vi "Close.vi"(8 "error in (no error)":errorcluster, 11 "CSV in":refnum<class "CSV.lvclass">) -> (0 "error out":errorcluster, 3 "CSV out":refnum<class "CSV.lvclass">)   [LabVIEW 2014, in "CSV.lvclass"]
uses:
  CSV.lvclass
  Report/Report.lvclass
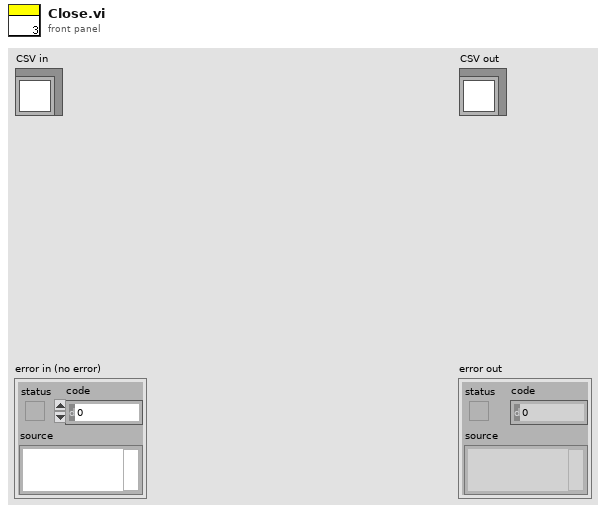
[diagram p1: front panel]
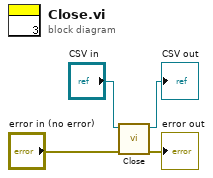
[diagram p0: block diagram]
diagram:
  n1 = call-parent "Close.vi"("error in (no error)"="error in (no error)", "Report in"="CSV in") -> ("error out"=→"error out":errorcluster, "Report out"=→"CSV out":refnum<class "CSV.lvclass">)  [unwired: 8 in]
